vi "calc_pixelhits.vi"(8 "error in":errorcluster, 9 "Smooth_coeffs_cluster":T1 {"Coeff 1" min=0.0 max=1.0 step=0.05; "Coeff 2" min=0.0 max=1.0 step=0.05}, 10 "Lookup arrays":T2, 11 "Pixelhits array in":refnum<data-value>) -> (0 "error out":errorcluster, 3 "Pixelhits array out":refnum<data-value>)   [LabVIEW 2011, in "Fiberscope_library.lvlib"]
uses:
  Fiberscope_library.lvlib
  typedefs/lookup_arrays_ref_cluster.ctl
  typedefs/smooth_coeffs_cluster.ctl
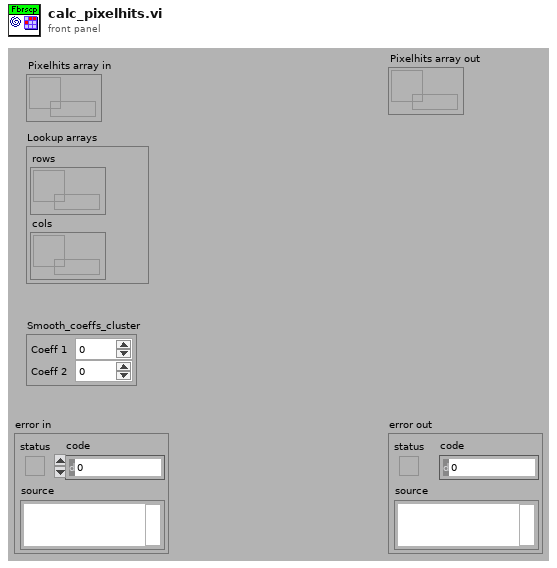
[diagram p1: front panel]
types:
  T1 = typedef "Fiberscope_library.lvlib/smooth_coeffs_cluster.ctl" = cluster{"Coeff 1":dbl, "Coeff 2":dbl}
  T2 = typedef "Fiberscope_library.lvlib/lookup_arrays_ref_cluster.ctl" = cluster{"rows":refnum<data-value>, "cols":refnum<data-value>}
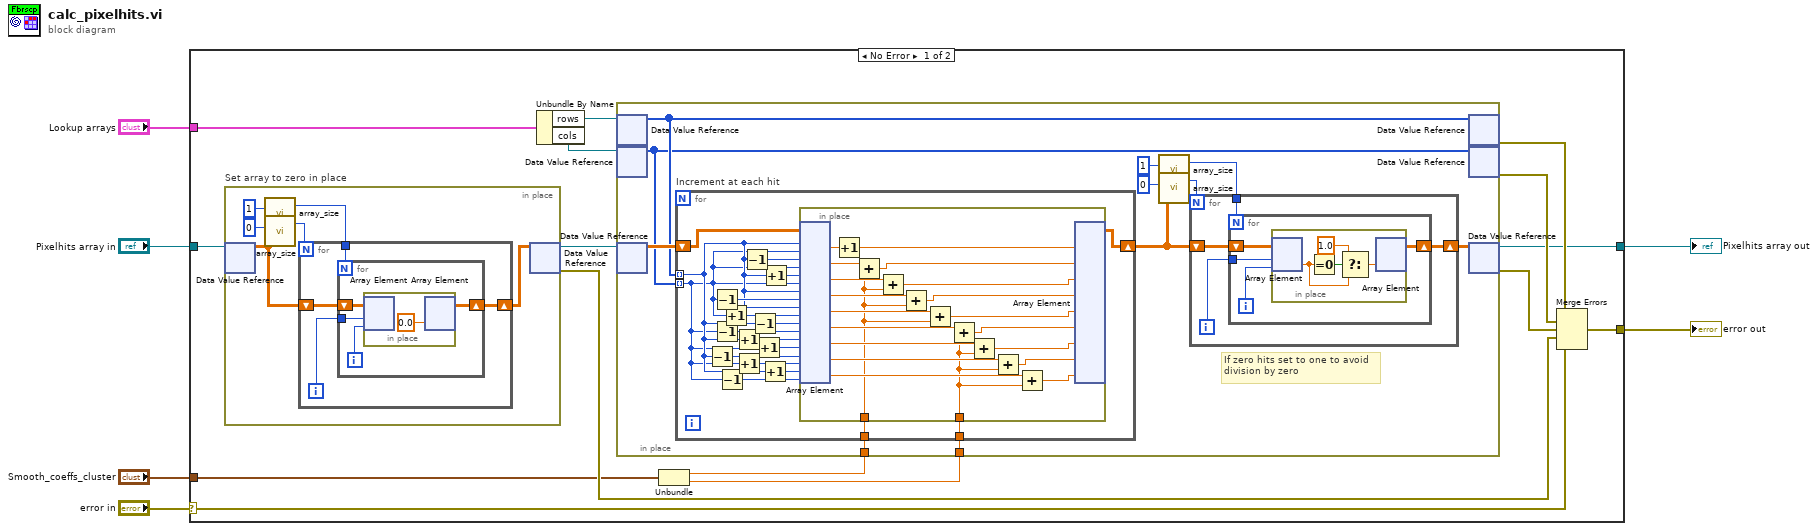
[diagram p0: block diagram]
diagram:
  n1 = case shown="No Error" "error in" {
    selector: "error in" -> [w10 w99]
    tunnel: [w13 w99] -> w5
    tunnel: [w12 w98] -> w3
    tunnel: "Pixelhits array in" -> [w11 w98]
    tunnel: "Lookup arrays" -> [w21 _]
    tunnel: "Smooth_coeffs_cluster" -> [w9 _]
    frame No Error {
      n2 = in-place "Set array to zero in place" {
        n3 = in-place-dvr #1(w11) -> (w24:dbl[][])  [unwired: 1 out]
        n4 = call "array_size.vi"("Array"=w24, "Dimension"=1) -> ("Dimension size"=w22:i32)  [unwired: 4 in]
        n5 = call "array_size.vi"("Array"=w24, "Dimension"=0) -> ("Dimension size"=w25:i32)  [unwired: 4 in]
        n6 = for {
          N: w25 -> [_]
          shift-right: [w29] -> w27
          shift-left: w24 -> [w31]
          tunnel: w22 -> [w28]
          i -> [w30]
          n7 = for {
            N: w28 -> [_]
            shift-right: [w32] -> w29
            shift-left: w31 -> [w35]
            tunnel: w30 -> [w34]
            i -> [w33]
            n8 = in-place {
              n9 = in-place-array #2(w35, w34, w33) -> ()  [unwired: 1 out]
              n10 = in-place-array #2(0.0 ("element")) -> (w32:dbl[][])  [unwired: 2 out]
            }
          }
        }
        n11 = in-place-dvr #1(w27) -> (w18:refnum<data-value>, w14:errorcluster)
      }
      n12 = Unbundle By Name(w21) -> ("rows"=w20:refnum<data-value>, "cols"=w19:refnum<data-value>)
      n13 = Unbundle(w9) -> ("Coeff 1"=w8:dbl, "Coeff 2"=w7:dbl)
      n14 = in-place {
        in-place-border: w8 -> [w38]
        in-place-border: w7 -> [w37]
        # "If zero hits set to one to avoid\ndivision by zero"
        n15 = in-place-dvr #3(w20) -> (w46:i32[])  [unwired: 1 out]
        n16 = in-place-dvr #4(w19) -> (w45:i32[])  [unwired: 1 out]
        n17 = in-place-dvr #5(w18) -> (w47:dbl[][])  [unwired: 1 out]
        n18 = for "Increment at each hit" {
          shift-right: [w64] -> w41
          shift-left: w47 -> [w73]
          tunnel: w45 -> [w66] mode=indexing
          tunnel: w46 -> [w72] mode=indexing
          tunnel: w38 -> [w61]
          tunnel: w37 -> [w60]
          n19 = Decrement(x=w72) -> (x-1=w69:i32)
          n20 = Decrement(x=w66) -> (x-1=w74:i32)
          n21 = Decrement(x=w66) -> (x-1=w76:i32)
          n22 = Decrement(x=w66) -> (x-1=w77:i32)
          n23 = Increment(x=w66) -> (x+1=w75:i32)
          n24 = Increment(x=w72) -> (x+1=w67:i32)
          n25 = Increment(x=w66) -> (x+1=w70:i32)
          n26 = Decrement(x=w72) -> (x-1=w62:i32)
          n27 = Decrement(x=w72) -> (x-1=w65:i32)
          n28 = Increment(x=w66) -> (x+1=w68:i32)
          n29 = Increment(x=w72) -> (x+1=w71:i32)
          n30 = Increment(x=w72) -> (x+1=w63:i32)
          n31 = in-place {
            in-place-border: w61 -> [w79]
            in-place-border: w60 -> [w78]
            n32 = in-place-array #6(w73, w72, w66, w62, w66, w63, w66, w72, w74, w72, w75, w65, w76, w67, w68, w69, w70, w71, w77) -> (w97:dbl, w95:dbl, w94:dbl, w93:dbl, w92:dbl, w91:dbl, w90:dbl, w89:dbl, w88:dbl)
            n33 = Increment(x=w97) -> (x+1=w96:dbl)
            n34 = Add(x=w95, y=w79) -> (x+y=w87:dbl)
            n35 = Add(x=w94, y=w79) -> (x+y=w86:dbl)
            n36 = Add(x=w93, y=w79) -> (x+y=w85:dbl)
            n37 = Add(x=w92, y=w79) -> (x+y=w84:dbl)
            n38 = Add(x=w91, y=w78) -> (x+y=w83:dbl)
            n39 = Add(x=w90, y=w78) -> (x+y=w82:dbl)
            n40 = Add(x=w89, y=w78) -> (x+y=w81:dbl)
            n41 = Add(x=w88, y=w78) -> (x+y=w80:dbl)
            n42 = in-place-array #6(w96, w87, w86, w85, w84, w83, w82, w81, w80) -> (w64:dbl[][])  [unwired: 18 out]
          }
        }
        n43 = call "array_size.vi"("Array"=w41, "Dimension"=1) -> ("Dimension size"=w40:i32)  [unwired: 4 in]
        n44 = call "array_size.vi"("Array"=w41, "Dimension"=0) -> ("Dimension size"=w39:i32)  [unwired: 4 in]
        n45 = for {
          N: w39 -> [_]
          shift-right: [w49] -> w44
          shift-left: w41 -> [w51]
          tunnel: w40 -> [w48]
          i -> [w50]
          n46 = for {
            N: w48 -> [_]
            shift-right: [w52] -> w49
            shift-left: w51 -> [w55]
            tunnel: w50 -> [w54]
            i -> [w53]
            n47 = in-place {
              n48 = in-place-array #7(w55, w54, w53) -> (w58:dbl)
              n49 = Equal To 0?(x=w58) -> (x = 0?=w59:bool)
              n50 = Select(t=1.0, s=w59, f=w58) -> (s? t:f=w56:dbl)
              n51 = in-place-array #7(w56) -> (w52:dbl[][])  [unwired: 2 out]
            }
          }
        }
        n52 = in-place-dvr #3(w46) -> (w17:errorcluster)  [unwired: 1 out]
        n53 = in-place-dvr #4(w45) -> (w16:errorcluster)  [unwired: 1 out]
        n54 = in-place-dvr #5(w44) -> (w12:refnum<data-value>, w15:errorcluster)
      }
      n55 = Merge Errors(w17, w16, w15, w14, w10) -> (w13:errorcluster)
    }
    frame Error {
    }
  }
  "error out" <- w5
  "Pixelhits array out" <- w3
